vi "Sensor Test Controller.vi"(8 "error in":errorcluster) -> ()   [LabVIEW 2019]
doc: "This VI executes continuously carrying out the current operation and responding to updates or new operations. It will often contain the timing or control code that is difficult to place directly in TeleOp. This VI generally opens all sensors and motors and isolates the rest of the robot code from knowing how the operations are carried out."
uses:
  <vilib>/Rock Robotics/WPI/Framework/Completion Status.ctl
  Sensor Test Setpoints.ctl
  Sensor Test Operations.ctl
  <vilib>/Rock Robotics/Network Tables/NT Read Number.vi
  <vilib>/Rock Robotics/Network Tables/NT Write Boolean.vi
panel:
  in  "Interactive Values":T1
  out "Current\nCmd":string
  in  "Buttons":cluster{"Execute Cmd":bool, "Abort Cmd":bool}
  out "Command Timing":cluster{"Start Time (ms)":u32, "Iterations":i32}
  out "Status":T3
  # "Tip: It may be helpful to observe inputs and sensor values.\nYou may also want to display tuning or debugging controls."
  # "Interactive Command: You may fill in the settings for a command\nand schedule it with the Execute button. You can observe and abort\nany command while fine tuning the code for the controller."
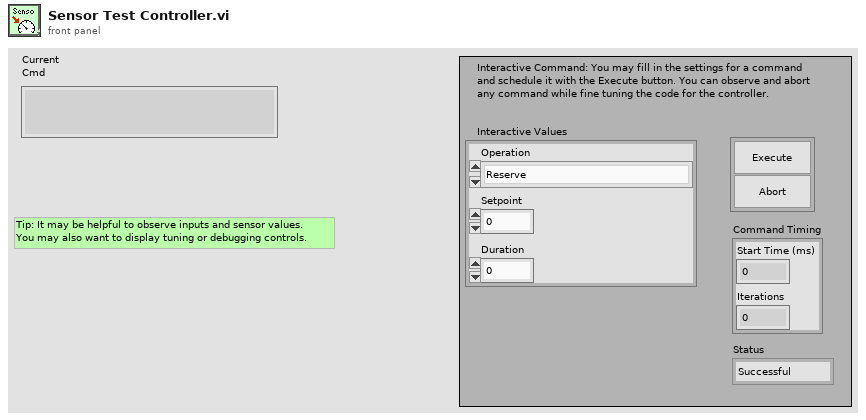
[diagram p1: front panel]
types:
  T1 = typedef "Sensor Test Setpoints.ctl" = cluster{"Operation":T2, "Setpoint":dbl, "Duration":dbl}
  T2 = typedef "Sensor Test Operations.ctl" = enum16{"Reserve", "Read Current", "Immediate", "Limelight Control", "Navx Control"}
  T3 = typedef "Completion Status.ctl" = enum16{"Successful", "Aborted", "Incomplete"}
  T4 = typedef "Command Status Info.ctl" = cluster{"Name":string, "Status":T3, "notifier out":T5}
  T5 = typedef "Completion Notifier.ctl" = refnum<notifier>
  T6 = cluster{"Current Command":T1, "Command Timing":cluster{"Start Time (ms)":u32, "Iterations":i32}, "Command Arguments":cluster{"Command Info":T4, "Description":string, "Default Command":T1, "queue out":refnum<queue>, "Subsystem Name":string}}
  T7 = typedef "WPI_MotorControlDeviceRef.ctl" = cluster{"DeviceStatus":errorcluster, "Type":T8, "PWM":cluster{"PWM Channel":T9, "DeadBand":T10}, "CAN":cluster{"Device Number":u8, "SetOutput VI Ref":variant, "GetOutput VI Ref":variant, "Enable VI Ref":variant, "Disable VI Ref":variant, "Data":variant}, "Invert":bool, "DIO PWM":cluster{"PWM \"Enable\" Channel":T9, "DIOChannel":T11, "PWM Rate":dbl}}
  T8 = typedef "WPI_MotorControlType.ctl" = enum16{"PWM", "CAN", "DIO PWM"}
  T9 = typedef "FPGA_DIOPWMChannel.ctl" = enum8{"PWM 0", "PWM 1", "PWM 2", "PWM 3", "PWM 4", "PWM 5", "PWM 6", "PWM 7", "PWM 8", "PWM 9", "PWM MXP 0", "PWM MXP 1", "PWM MXP 2", "PWM MXP 3", "PWM MXP 4", "PWM MXP 5", "PWM MXP 6", "PWM MXP 7", "PWM MXP 8", "PWM MXP 9", "Invalid"}
  T10 = typedef "WPI_PWMDeadband.ctl" = cluster{"Name":string, "maxPositivePwm":i32, "minPositivePwm":i32, "centerPwm":i32, "maxNegativePwm":i32, "minNegativePwm":i32, "angularRange":u16}
  T11 = typedef "FPGA_DIOChannel.ctl" = enum8{"DIO 0", "DIO 1", "DIO 2", "DIO 3", "DIO 4", "DIO 5", "DIO 6", "DIO 7", "DIO 8", "DIO 9", "DIO MXP 0", "DIO MXP 1", "DIO MXP 2", "DIO MXP 3", "DIO MXP 4", "DIO MXP 5", "DIO MXP 6", "DIO MXP 7", "DIO MXP 8", "DIO MXP 9", "DIO MXP 10", "DIO MXP 11", "DIO MXP 12", "DIO MXP 13", "DIO MXP 14", "DIO MXP 15", "SPI Port CS1", "SPI Port CS2", "SPI Port CS3", "SPI Port MISO", "SPI Port MOSI", "Invalid"}
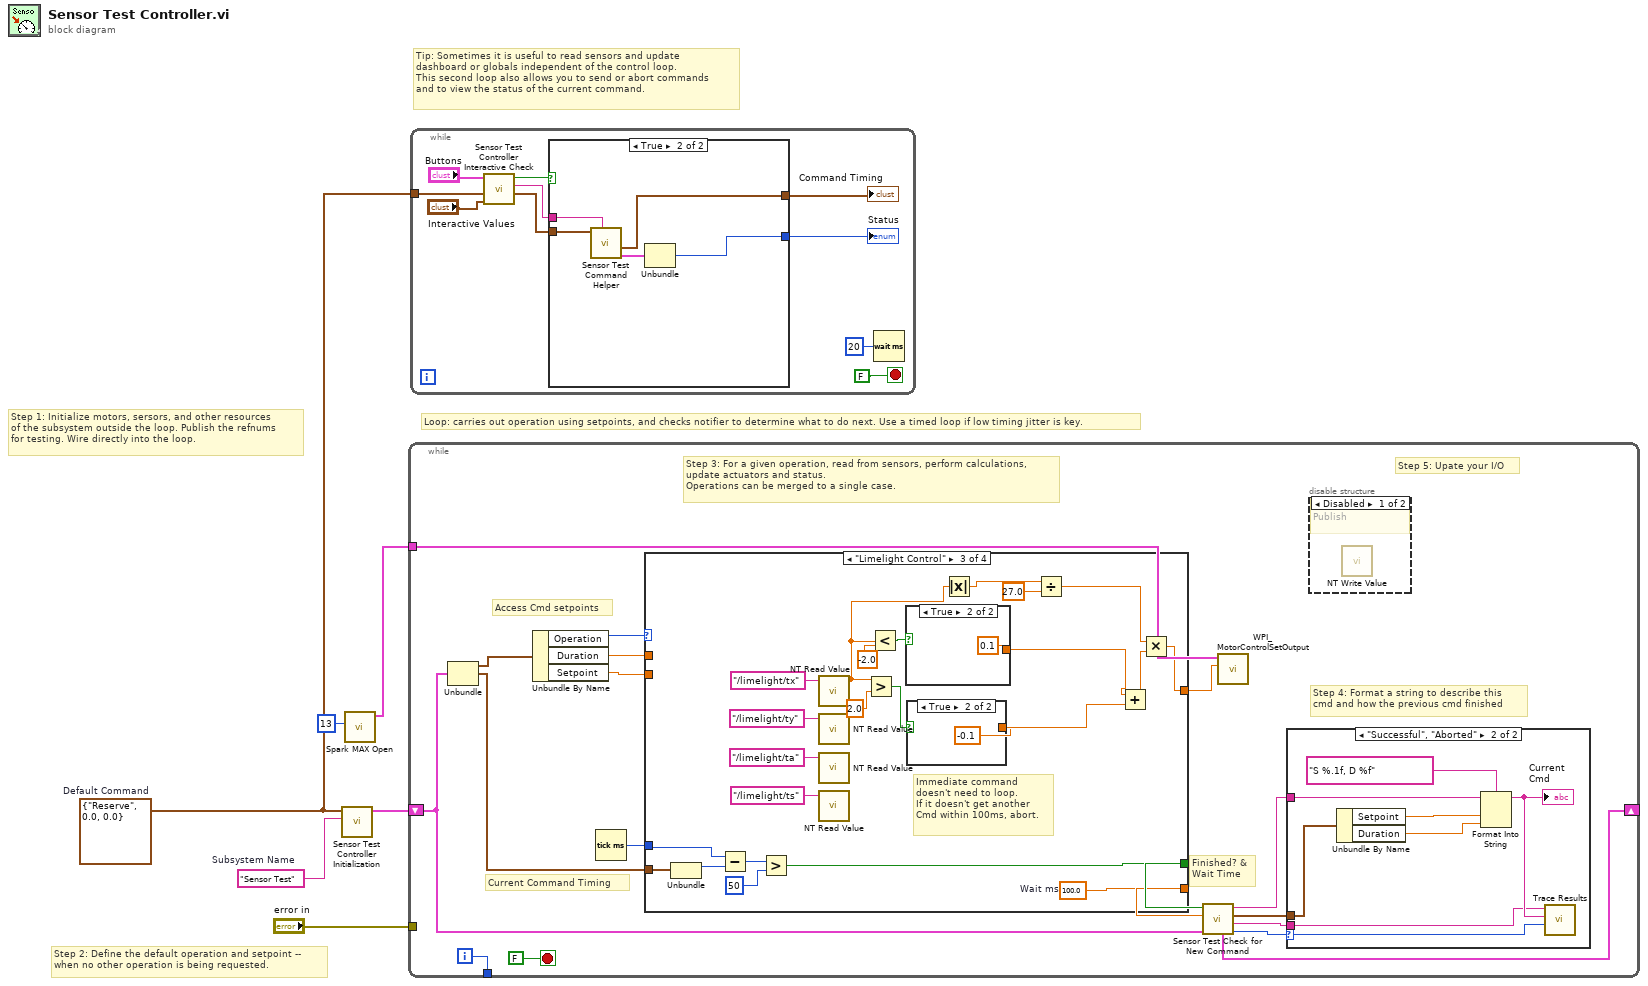
[diagram p0: block diagram]
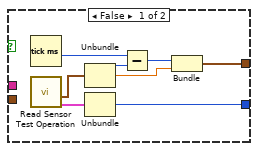
[diagram p2: hidden frame]
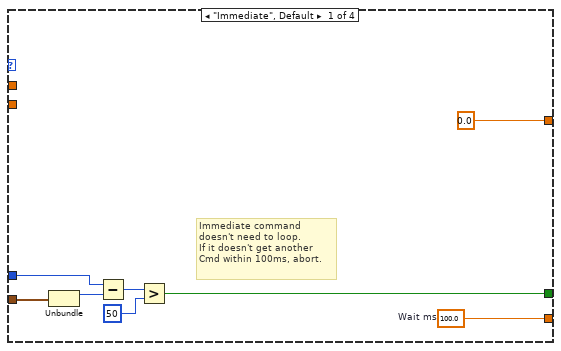
[diagram p5: hidden frame]
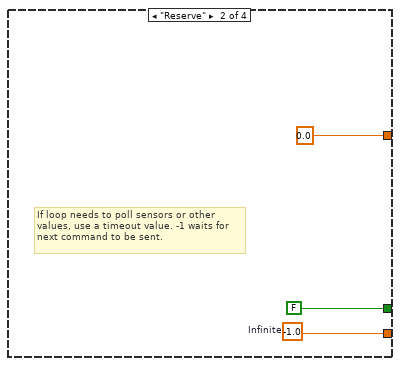
[diagram p6: hidden frame]
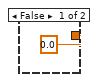
[diagram p7: hidden frame]
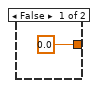
[diagram p8: hidden frame]
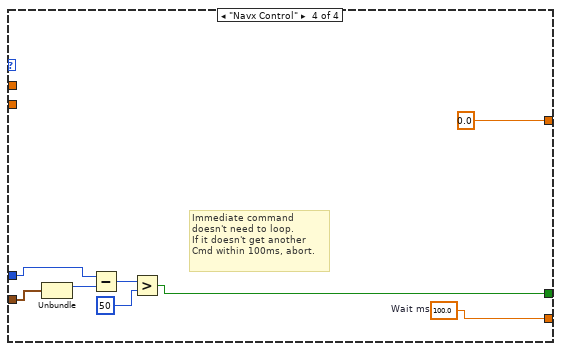
[diagram p9: hidden frame]
diagram:
  w3 = T1 {"Operation"=enum."Reserve", "Setpoint"=0.0, "Duration"=0.0}  # Default Command
  w4 = "Sensor Test"  # Subsystem Name
  # "Tip: Sometimes it is useful to read sensors and update\ndashboard or globals independent of the control loop.\nThis second loop also allows you to send or abort commands\nand to view the status of the current command."
  # "Step 2: Define the default operation and setpoint --\nwhen no other operation is being requested."
  # "Step 1: Initialize motors, sersors, and other resources\nof the subsystem outside the loop. Publish the refnums\nfor testing. Wire directly into the loop."
  # "Loop: carries out operation using setpoints, and checks notifier to determine what to do next. Use a timed loop if low timing jitter is key."
  n1 = call "Sensor Test Controller Initialization.vi"("Subsystem Name"=w4, "Default Command"=w3) -> ("Current Command"=w5:T6)  [unwired: 9 in]
  n2 = call <vilib>:"Spark MAX Open.vi"("Device Number"=u8 13) -> ("MotorControlDeviceRef"=w1:T7)  [unwired: 9 in, 1 out]
  n3 = while {
    shift-right: [w16] -> _
    shift-left: w5 -> [w9]
    tunnel: [w23] -> _
    tunnel: "error in" -> [_]
    tunnel: w1 -> [w8]
    i -> [w23]
    stop <- FALSE stop-if-true
    # "Step 5: Upate your I/O"
    # "Step 4: Format a string to describe this\ncmd and how the previous cmd finished"
    # "Current Command Timing"
    # "Access Cmd setpoints"
    # "Finished? &\nWait Time"
    # "Step 3: For a given operation, read from sensors, perform calculations,\nupdate actuators and status.\nOperations can be merged to a single case."
    n4 = Unbundle(w9) -> ("Current Command"=w22:T1, "Command Timing"=w18:cluster{"Start Time (ms)":u32, "Iterations":i32})  [unwired: 1 out]
    n5 = Unbundle By Name(w22) -> ("Operation"=w21:T2, "Duration"=w20:dbl, "Setpoint"=w17:dbl)
    n6 = Tick Count (ms)() -> (millisecond timer value=w19:u32)
    n7 = case shown="\"Limelight Control\"" w21 {
      tunnel: [w40 w43 w56 w72] -> w14
      tunnel: [w34 FALSE ("ignore previous (F)") w57 w71] -> w15
      tunnel: w18 -> [w36 _ w59 w73]
      tunnel: w20 -> [_ _ _ _]
      tunnel: w19 -> [w35 _ w58 w74]
      tunnel: w17 -> [_ _ _ _]
      tunnel: [0.0 ("Output") 0.0 ("Output") w46 0.0 ("Output")] -> w7
      frame "Immediate", Default {
        w40 = 100.0  # Wait ms
        # "Immediate command\ndoesn't need to loop.\nIf it doesn't get another\nCmd within 100ms, abort."
        n8 = Unbundle(w36) -> ("Start Time (ms)"=w39:u32)  [unwired: 1 out]
        n9 = Subtract(x=w35, y=w39) -> (x-y=w38:u32)
        n10 = Greater?(x=w38, y=u8 50 ("Left Motor")) -> (0:w34:bool)
      }
      frame "Reserve" {
        w43 = -1.0  # Infinite
        # "If loop needs to poll sensors or other\nvalues, use a timeout value. -1 waits for\nnext command to be sent."
      }
      frame "Limelight Control" {
        w56 = 100.0  # Wait ms
        # "Immediate command\ndoesn't need to loop.\nIf it doesn't get another\nCmd within 100ms, abort."
        n11 = Unbundle(w59) -> ("Start Time (ms)"=w62:u32)  [unwired: 1 out]
        n12 = Subtract(x=w58, y=w62) -> (x-y=w61:u32)
        n13 = Greater?(x=w61, y=u8 50 ("Left Motor")) -> (0:w57:bool)
        n14 = call-poly <vilib>:"NT Read Value.vi"("Name"="/limelight/tx") -> ("Numeric"=w49:dbl)  [unwired: 9 in, 1 out]
        n15 = call-poly <vilib>:"NT Read Value.vi"("Name"="/limelight/ty") -> ()  [unwired: 9 in, 2 out]
        n16 = call-poly <vilib>:"NT Read Value.vi"("Name"="/limelight/ta") -> ()  [unwired: 9 in, 2 out]
        n17 = call-poly <vilib>:"NT Read Value.vi"("Name"="/limelight/ts") -> ()  [unwired: 9 in, 2 out]
        n18 = Greater?(x=w49, y=2.0) -> (0:w52:bool)
        n19 = Less?(x=w49, y=-2.0) -> (x < y?=w53:bool)
        n20 = case shown="True" w53 {
          tunnel: [0.0 ("Output") 0.1 ("Output")] -> w51
          frame False {
          }
          frame True {
          }
        }
        n21 = case shown="True" w52 {
          tunnel: [0.0 ("Output") -0.1 ("Output")] -> w50
          frame False {
          }
          frame True {
          }
        }
        n22 = Absolute Value(x=w49) -> (abs(x)=w48:dbl)
        n23 = Divide(x=w48, y=27.0) -> (x/y=w45:dbl)
        n24 = Add(x=w51, y=w50) -> (x+y=w44:dbl)
        n25 = Multiply(x=w45, y=w44) -> (x*y=w46:dbl)
      }
      frame "Navx Control" {
        w72 = 100.0  # Wait ms
        # "Immediate command\ndoesn't need to loop.\nIf it doesn't get another\nCmd within 100ms, abort."
        n26 = Unbundle(w73) -> ("Start Time (ms)"=w76:u32)  [unwired: 1 out]
        n27 = Subtract(x=w74, y=w76) -> (x-y=w77:u32)
        n28 = Greater?(x=w77, y=u8 50 ("Left Motor")) -> (0:w71:bool)
      }
    }
    n29 = call "Sensor Test Check for New Command.vi"("Current Command"=w9, "Wait time (ms)"=w14, "Finished?"=w15) -> ("Completion"=w10:T3, "Subsystem Name"=w11:string, "Current Command"=w12:T1, "Initial Trace String"=w13:string, "NextCommand"=w16:T6)  [unwired: 4 in]
    n30 = call <vilib>:"WPI_MotorControlSetOutput.vi"("Output"=w7, "MotorControlDevRef"=w8) -> ()  [unwired: 7 in, 3 out]
    n31 = case shown="\"Successful\", \"Aborted\"" w10 {
      selector: w10 -> [_ w32]
      tunnel: w13 -> [_ w28]
      tunnel: w12 -> [_ w29]
      tunnel: w11 -> [_ w25]
      frame "Incomplete", Default {
        # "Continuing current command"
      }
      frame "Successful", "Aborted" {
        # "Report and setup for next command"
        n32 = Unbundle By Name(w29) -> ("Setpoint"=w31:dbl, "Duration"=w26:dbl)
        n33 = Format Into String(format string="S %.1f, D %f", initial string=w28, w31, w26) -> (resulting string=w27:string)  [unwired: 1 in, 1 out]
        "Current\nCmd" <- w27
        n34 = call <vilib>:"Trace Results.vi"("Status of previous command"=w32, "Description"=w27, "Subsystem"=w25) -> ()  [unwired: 9 in]
      }
    }
    n35 = disable-structure shown="Disabled" {
      frame Disabled {
        # "Publish"
        n36 = call-poly <vilib>:"NT Write Value.vi"() -> ()  [unwired: 11 in, 1 out]
      }
      frame Enabled {
      }
    }
  }
  n37 = while {
    tunnel: w3 -> [w85]
    stop <- FALSE stop-if-true
    n38 = call "Sensor Test Controller Interactive Check.vi"("Interactive Command in"="Interactive Values", "Default Command"=w85, "Buttons"="Buttons") -> ("Interactive Command out"=w82:T1, "Trace String"=w83:string, "Schedule"=w84:bool)  [unwired: 6 in]
    n39 = case shown="True" w84 {
      tunnel: [w96 w101] -> w81
      tunnel: w82 -> [_ w99]
      tunnel: [w92 w97] -> w80
      tunnel: w83 -> [_ w100]
      frame False {
        n40 = Tick Count (ms)() -> (millisecond timer value=w91:u32)
        n41 = call "Read Sensor Test Operation.vi"() -> ("Command Info"=w89:T4, "SubSystem Data"=w90:T1)  [unwired: 9 in, 1 out]
        n42 = Unbundle(w90) -> ("Operation"=w95:T2, "Setpoint"=w93:dbl)  [unwired: 1 out]
        n43 = Unbundle(w89) -> ("Status"=w96:T3)  [unwired: 2 out]
        n44 = Subtract(x=w91, y=w95) -> (x-y=w94:u32)
        n45 = Bundle(w94, "Setpoint"=w93) -> (w92:cluster{u32, "Setpoint":dbl})  [unwired: 1 in]
      }
      frame True {
        n46 = call "Sensor Test Command Helper.vi"("Description"=w100, "SubSystem Data"=w99) -> ("Command Info Out"=w98:T4, "Command Timing"=w97:cluster{"Start Time (ms)":u32, "Iterations":i32})  [unwired: 7 in, 1 out]
        n47 = Unbundle(w98) -> ("Status"=w101:T3)  [unwired: 2 out]
      }
    }
    "Status" <- w81
    "Command Timing" <- w80
    n48 = Wait (ms)(milliseconds to wait=u32 20) -> ()  [unwired: 1 out]
  }
